vi "Insight Initialize.vi"(2 "Digital Module":T1) -> ()   [LabVIEW 2015]
uses:
  <vilib>/Rock Robotics/SystemInterfaces/Typedef/FPGA_TypedefDigitalModule.ctl
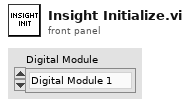
[diagram p1: front panel]
types:
  T1 = typedef "FPGA_TypedefDigitalModule.ctl" = enum16{"Digital Module 1", "Digital Module 2"}
  T2 = typedef "WPI_I2CDevRef.ctl" = cluster{"DevStatus":errorcluster, "Digital Module":T1, "Device Address":u8}
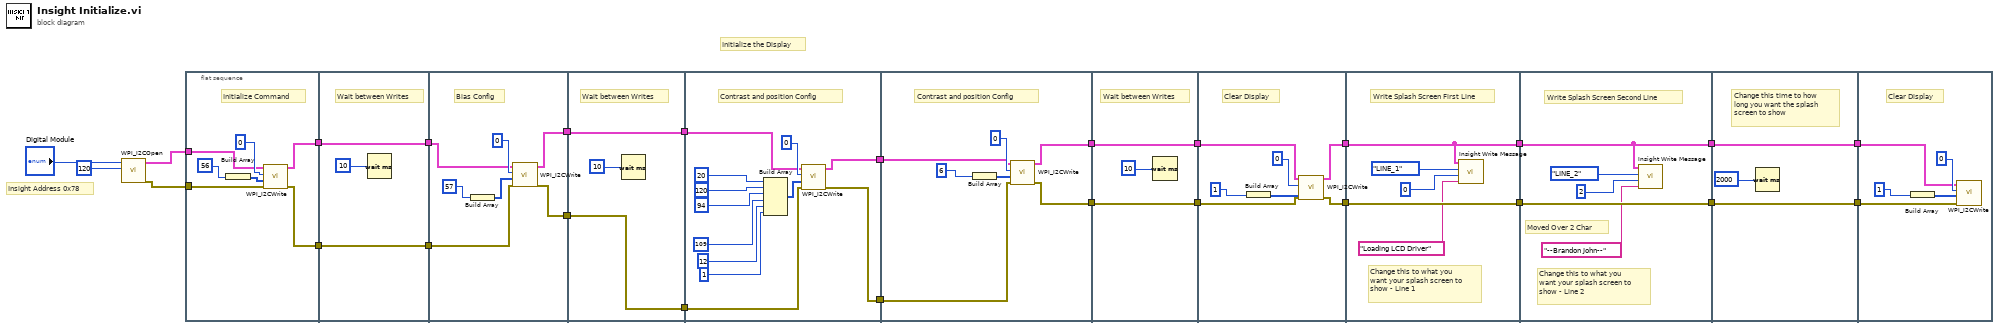
[diagram p0: block diagram]
diagram:
  # "Initialize the Display"
  # "Insight Address 0x78"
  n1 = call <vilib>:"WPI_I2COpen.vi"("Device Address"=u8 120, "Digital Module (Module 1)"="Digital Module") -> ("error out"=w1:errorcluster, "I2CDevRef"=w2:T2)  [unwired: 8 in]
  n2 = flat-sequence {
    tunnel: [w30] -> w24
    tunnel: [w29] -> w23
    tunnel: w2 -> [w28]
    tunnel: w1 -> [w27]
    tunnel: [w35] -> w22
    tunnel: w24 -> [w35]
    tunnel: [w34] -> w21
    tunnel: w23 -> [w34]
    tunnel: w22 -> [w42]
    tunnel: w21 -> [w41]
    tunnel: [w40] -> w20
    tunnel: [w39] -> w19
    tunnel: [w45] -> w18
    tunnel: w20 -> [w45]
    tunnel: w19 -> [w44]
    tunnel: [w44] -> w17
    tunnel: w18 -> [w57]
    tunnel: w17 -> [w56]
    tunnel: [w48] -> w16
    tunnel: [w47] -> w15
    tunnel: w16 -> [w62]
    tunnel: w15 -> [w61]
    tunnel: [w60] -> w14
    tunnel: [w59] -> w13
    tunnel: [w67] -> w12
    tunnel: w14 -> [w67]
    tunnel: [w66] -> w11
    tunnel: w13 -> [w66]
    tunnel: w12 -> [w69]
    tunnel: [w70] -> w10
    tunnel: w11 -> [w72]
    tunnel: [w71] -> w9
    tunnel: w10 -> [w80]
    tunnel: [w80] -> w8
    tunnel: w9 -> [w76]
    tunnel: [w76] -> w7
    tunnel: w8 -> [w85]
    tunnel: [w85] -> w6
    tunnel: w7 -> [w81]
    tunnel: [w81] -> w5
    tunnel: w6 -> [w88]
    tunnel: [w88] -> w4
    tunnel: w5 -> [w87]
    tunnel: [w87] -> w3
    tunnel: w4 -> [w92]
    tunnel: w3 -> [w91]
    frame #0 {
      # "Initialize Command"
      n3 = Build Array(u8 56 ("Device Address")) -> (w31:u8[])
      n4 = call <vilib>:"WPI_I2CWrite.vi"("error in (no error)"=w27, "I2CDataToSend"=w31, "I2CRegister"=u8 0, "I2CDevRef"=w28) -> ("error out"=w29:errorcluster, "I2CDevRef"=w30:T2)  [unwired: 6 in]
    }
    frame #1 {
      # "Wait between Writes"
      n5 = Wait (ms)(milliseconds to wait=u32 10) -> ()  [unwired: 1 out]
    }
    frame #2 {
      # "Bias Config"
      n6 = Build Array(u8 57 ("Device Address")) -> (w37:u8[])
      n7 = call <vilib>:"WPI_I2CWrite.vi"("error in (no error)"=w41, "I2CDataToSend"=w37, "I2CRegister"=u8 0, "I2CDevRef"=w42) -> ("error out"=w39:errorcluster, "I2CDevRef"=w40:T2)  [unwired: 6 in]
    }
    frame #3 {
      # "Wait between Writes"
      n8 = Wait (ms)(milliseconds to wait=u32 10) -> ()  [unwired: 1 out]
    }
    frame #4 {
      # "Contrast and position Config"
      n9 = Build Array(u8 20 ("Device Address"), u8 120 ("Device Address"), u8 94 ("Device Address"), u8 109 ("Device Address"), u8 12 ("Device Address"), u8 1 ("Device Address")) -> (w52:u8[])
      n10 = call <vilib>:"WPI_I2CWrite.vi"("error in (no error)"=w56, "I2CDataToSend"=w52, "I2CRegister"=u8 0, "I2CDevRef"=w57) -> ("error out"=w47:errorcluster, "I2CDevRef"=w48:T2)  [unwired: 6 in]
    }
    frame #5 {
      # "Contrast and position Config"
      n11 = Build Array(u8 6 ("Device Address")) -> (w65:u8[])
      n12 = call <vilib>:"WPI_I2CWrite.vi"("error in (no error)"=w61, "I2CDataToSend"=w65, "I2CRegister"=u8 0, "I2CDevRef"=w62) -> ("error out"=w60:errorcluster, "I2CDevRef"=w59:T2)  [unwired: 6 in]
    }
    frame #6 {
      # "Wait between Writes"
      n13 = Wait (ms)(milliseconds to wait=u32 10) -> ()  [unwired: 1 out]
    }
    frame #7 {
      # "Clear Display"
      n14 = Build Array(u8 1 ("Device Address")) -> (w74:u8[])
      n15 = call <vilib>:"WPI_I2CWrite.vi"("error in (no error)"=w69, "I2CDataToSend"=w74, "I2CRegister"=u8 0, "I2CDevRef"=w72) -> ("error out"=w70:errorcluster, "I2CDevRef"=w71:T2)  [unwired: 6 in]
    }
    frame #8 {
      # "Change this to what you \nwant your splash screen to\nshow - Line 1"
      # "Write Splash Screen First Line"
      n16 = call "Insight Write Message.vi"("User Data"="Loading LCD Driver", "Position"=u8 0, "Line"=enum16{"LINE_1", "LINE_2"}."LINE_1", "I2CDevRef"=w76) -> ()  [unwired: 1 in]
    }
    frame #9 {
      # "Write Splash Screen Second Line"
      # "Change this to what you \nwant your splash screen to\nshow - Line 2"
      # "Moved Over 2 Char"
      n17 = call "Insight Write Message.vi"("User Data"="--Brandon John--", "Position"=u8 2, "Line"=enum16{"LINE_1", "LINE_2"}."LINE_2", "I2CDevRef"=w81) -> ()  [unwired: 1 in]
    }
    frame #10 {
      # "Change this time to how \nlong you want the splash\nscreen to show"
      n18 = Wait (ms)(milliseconds to wait=u32 2000) -> ()  [unwired: 1 out]
    }
    frame #11 {
      # "Clear Display"
      n19 = Build Array(u8 1 ("Device Address")) -> (w90:u8[])
      n20 = call <vilib>:"WPI_I2CWrite.vi"("error in (no error)"=w92, "I2CDataToSend"=w90, "I2CRegister"=u8 0, "I2CDevRef"=w91) -> ()  [unwired: 6 in, 2 out]
    }
  }
